vi "Read File Path.vi"(8 "error in":errorcluster, 11 "JSON in":refnum<class "JSON.lvclass">) -> (0 "error out":errorcluster, 2 "File Path":path, 3 "JSON out":refnum<class "JSON.lvclass">)   [LabVIEW 2017, in "Report_lib.lvlib" / "JSON.lvclass"]
uses:
  JSON.lvclass
  JSON.lvclass/JSON.ctl
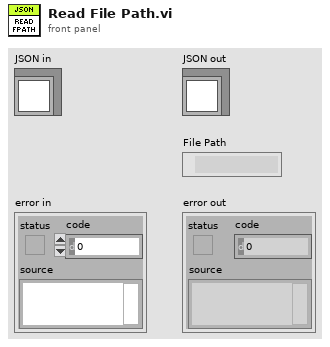
[diagram p1: front panel]
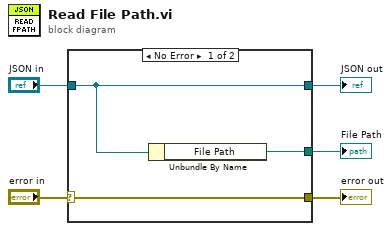
[diagram p0: block diagram]
diagram:
  n1 = case shown="No Error" "error in" {
    selector: "error in" -> [w8 w10]
    tunnel: [w8 w10] -> w4
    tunnel: [w7 w9] -> w2
    tunnel: "JSON in" -> [w7 w9]
    tunnel: [w6 _] -> w1
    frame No Error {
      n2 = Unbundle By Name(w7) -> ("File Path"=w6:path)
    }
    frame Error {
    }
  }
  "error out" <- w4
  "JSON out" <- w2
  "File Path" <- w1
